vi "Counter - Read multiple counters.vi"() -> ()   [LabVIEW 2020]
doc: "This example demonstrates how to use a counter input along with an external clock to continually sample the angular velocity measured from an encoder.\n\nFor instructions on how to connect your signals to the DAQ device, refer to your device documentation."
uses:
  <vilib>/Utility/error.llb/DialogType.ctl
  <vilib>/DAQmx/read.llb/DAQmx Read (Counter 1D U32 NChan 1Samp).vi
  <vilib>/DAQmx/create/channels.llb/DAQmx Create Channel (CI-Count Edges).vi
  <vilib>/DAQmx/configure/timing.llb/DAQmx Timing (Sample Clock).vi
  <vilib>/DAQmx/miscellaneous.llb/DAQmx Fill In Error Info.vi
  <resource>/objmgr/daqmx.rc
panel:
  out "Data":u32[](array[numeric])
  in  "Stop":bool
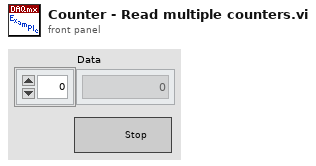
[diagram p1: front panel]
types:
  T1 = typedef "DialogType.ctl" = u16
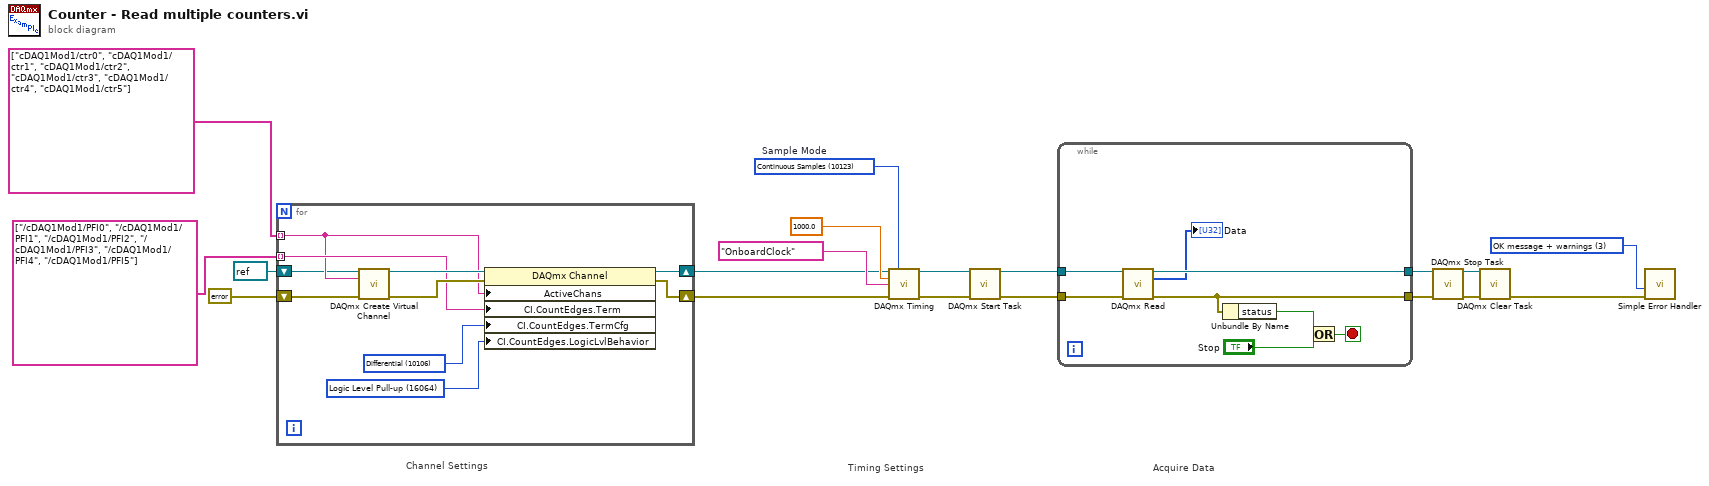
[diagram p0: block diagram]
diagram:
  w5 = T1 3 items=["no dialog", "OK message", "continue or stop message", "OK message + warnings", "continue/stop + warnings"] ("type of dialog (OK msg:1)")
  w19 = 10123 items=["Finite Samples"=10178, "Continuous Samples"=10123, "Hardware Timed Single Point"=12522]  # Sample Mode
  # "Acquire Data"
  # "Timing Settings"
  # "Channel Settings"
  n1 = for {
    tunnel: tag[] ["/cDAQ1Mod1/PFI0", "/cDAQ1Mod1/PFI1", "/cDAQ1Mod1/PFI2", "/cDAQ1Mod1/PFI3", "/cDAQ1Mod1/PFI4", "/cDAQ1Mod1/PFI5"] ("A Input Terminal") -> [w25] mode=indexing
    tunnel: tag[] ["cDAQ1Mod1/ctr0", "cDAQ1Mod1/ctr1", "cDAQ1Mod1/ctr2", "cDAQ1Mod1/ctr3", "cDAQ1Mod1/ctr4", "cDAQ1Mod1/ctr5"] ("Counter 1") -> [w24] mode=indexing
    shift-right: [w27] -> w11
    shift-left: refnum<k21> refnum ("task out") -> [w21]
    shift-right: [w26] -> w10
    shift-left: errorcluster {"status"=FALSE, "code"=0, "source"=""} ("error out") -> [w20]
    w22 = 16064 items=["Logic Level Pull-up"=16064, "None"=10230] ("CI.CountEdges.LogicLvlBehavior")
    w23 = 10106 items=["Differential"=10106, "RSE"=10083] ("CI.CountEdges.TermCfg")
    n2 = call-poly <vilib>:"DAQmx Create Virtual Channel.vi"("task in"=w21, "counter"=w24, "error in"=w20) -> ("task out"=w29:refnum<k21>, "error out"=w28:errorcluster)  [unwired: 11 in]
    n3 = property class="DAQmx Channel"(reference=w29, error in=w28, "ActiveChans"=w24, "CI.CountEdges.Term"=w25, "CI.CountEdges.TermCfg"=w23, "CI.CountEdges.LogicLvlBehavior"=w22) -> (reference out=w27:refnum<k21>, error out=w26:errorcluster)
  }
  n4 = call-poly <vilib>:"DAQmx Timing.vi"("task/channels in"=w11, "sample mode"=w19, "rate"=1000.0 ("Sample Rate"), "source"=tag "OnboardClock" ("Sample Clock Source"), "error in"=w10) -> ("task out"=w13:refnum<k21>, "error out"=w12:errorcluster)  [unwired: 9 in]
  n5 = call <vilib>:"DAQmx Start Task.vi"("task/channels in"=w13, "error in"=w12) -> ("task out"=w18:refnum<k21>, "error out"=w17:errorcluster)  [unwired: 12 in]
  n6 = while {
    tunnel: w18 -> [w37]
    tunnel: w17 -> [w36]
    tunnel: [w33] -> w8
    tunnel: [w34] -> w9
    stop <- w35 stop-if-true
    n7 = call-poly <vilib>:"DAQmx Read.vi"("task/channels in"=w37, "error in"=w36) -> ("task out"=w34:refnum<k21>, "data"=→"Data":u32[], "error out"=w33:errorcluster)  [unwired: 11 in]
    n8 = Unbundle By Name(w33) -> ("status"=w32:bool)
    n9 = Or(x=w32, y="Stop") -> (x .or. y?=w35:bool)
  }
  n10 = call <vilib>:"DAQmx Stop Task.vi"("task/channels in"=w9, "error in"=w8) -> ("task out"=w6:refnum<k21>, "error out"=w7:errorcluster)  [unwired: 12 in]
  n11 = call <vilib>:"DAQmx Clear Task.vi"("task in"=w6, "error in"=w7) -> ("error out"=w16:errorcluster)  [unwired: 13 in]
  n12 = call <vilib>:"Simple Error Handler.vi"("type of dialog (OK msg:1)"=w5, "error in (no error)"=w16) -> ()  [unwired: 3 in, 5 out]
